vi "Save_Portfolio.vi"(7 "Config File path":path caption="Config File Path", 8 "error in (no error)":errorcluster caption="entrée d'erreur (pas d'erreur)", 10 "path":path, 11 "Portfolio in":refnum<class "Portfolio.lvclass">) -> (0 "error out":errorcluster caption="sortie d'erreur", 3 "Portfolio en sortie":refnum<class "Portfolio.lvclass"> caption="DNL_LabVIEW Object out")   [LabVIEW 2012, in "Portfolio.lvclass"]
uses:
  Portfolio.lvclass
  Stock/Stock Parameters.ctl
  controls/Currencies.ctl
  Portfolio.lvclass/Portfolio.ctl
  Stock/Stock.lvclass/Stock.ctl
  Operations/Operations.lvclass
  Exchanges/Exchanges.lvclass
  <vilib>/Utility/config.llb/NI_LVConfig.lvlib
  Stock/Stock.lvclass
panel:
  in  "Stocks":T1[](array[typedef])
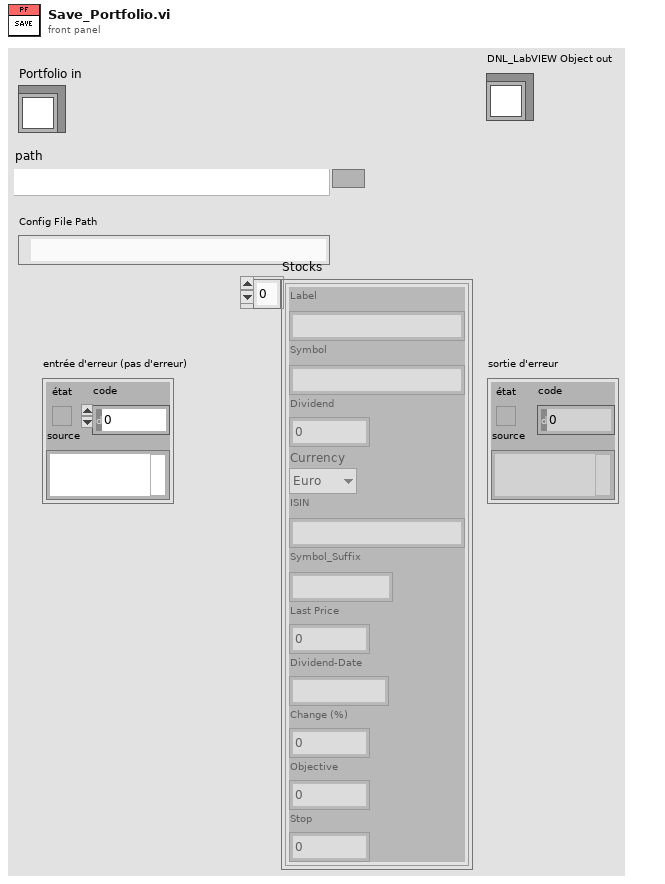
[diagram p1: front panel]
types:
  T1 = typedef "Stock.lvclass/Stock Parameters.ctl" = cluster{"Label":string, "Symbol":string, "Dividend":dbl, "Currency":T2, "ISIN":string, "Symbol_Suffix":string, "Last Price":dbl, "Dividend-Date":string, "Change (%)":dbl, "Objective":dbl, "Stop":dbl}
  T2 = typedef "Currencies.ctl" = enum16{"Euro", "Dollar", "Yen", "RIM", "CHF"}
  T3 = typedef "NI_LVConfig.lvlib/Config Data RefNum.ctl" = refnum<k1>
  T4 = typedef "Portfolio Parameters.ctl" = cluster{"Date":timestamp, "Name":string, "Cash":dbl, "Total":dbl, "Investissements":dbl, "Performance Totale (en %)":dbl, "Performance sur 1 an (en %)":dbl}
  T5 = typedef "Operation Parameters.ctl" = cluster{"Date":timestamp, "Operation Type":T6, "Amount":dbl, "Comment":string, "Currency":T2}
  T6 = typedef "Operation Type Enum.ctl" = enum16{"Coupons", "Dépot", "Retrait", "Intérêts", "Taxe"}
  T7 = typedef "Exchange Parameters.ctl" = cluster{"Date":timestamp, "Exchange Type":T8, "ISIN":string, "Label":string, "Price":dbl, "Qty":dbl, "Currency":T2, "Tax":dbl, "Comment":string, "PRU":dbl}
  T8 = typedef "Exchange.lvclass/Exchange Type Enum.ctl" = enum16{"ACHAT", "VENTE"}
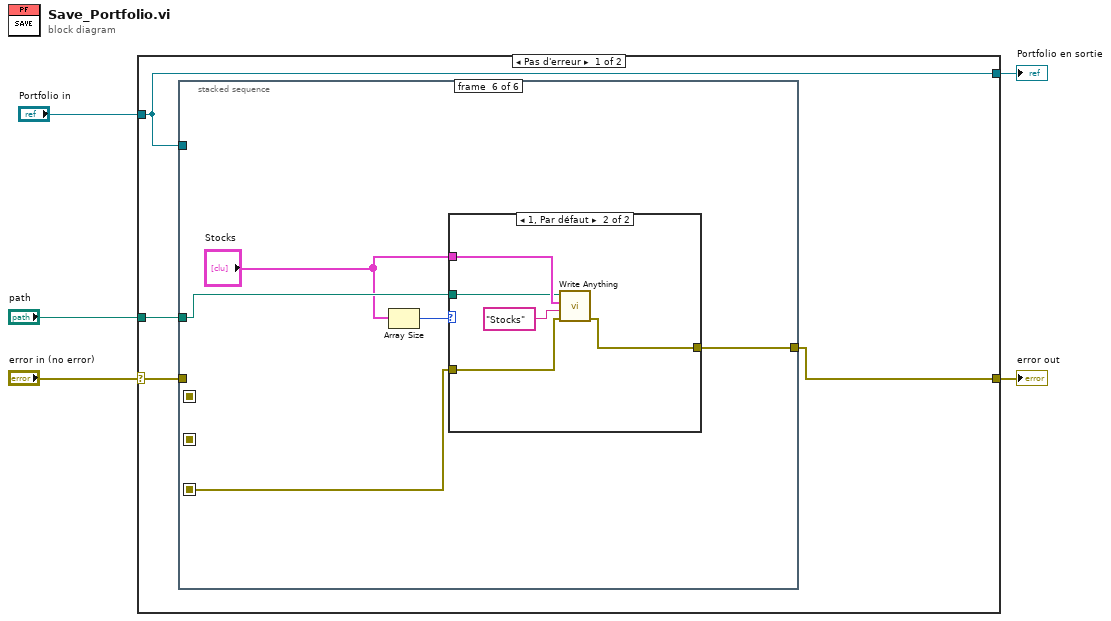
[diagram p0: block diagram]
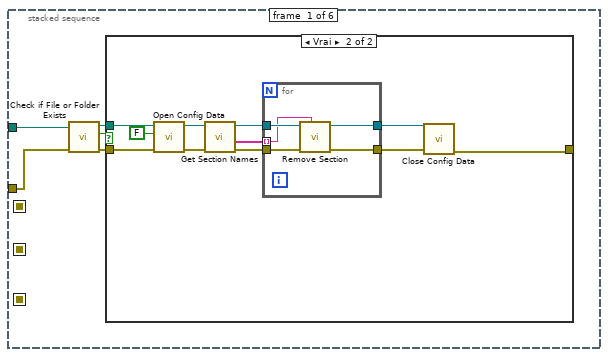
[diagram p2: hidden frame]
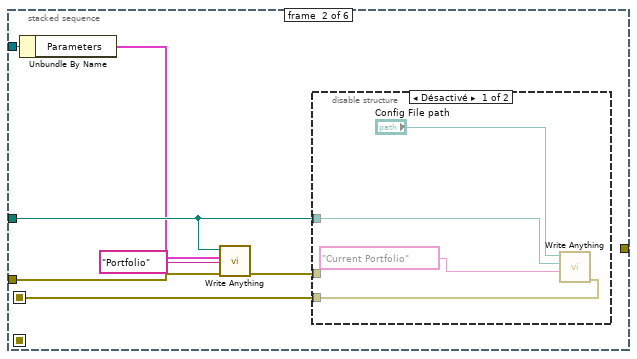
[diagram p4: hidden frame]
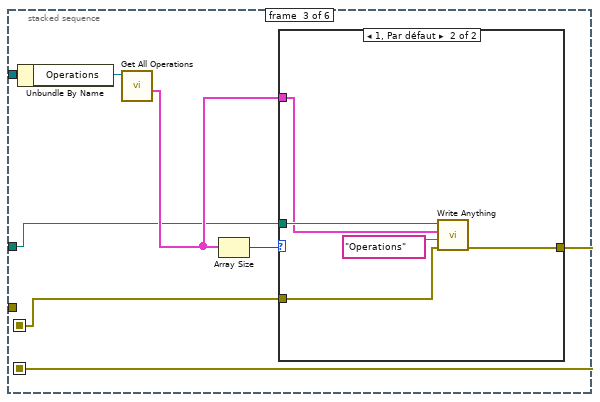
[diagram p6: hidden frame]
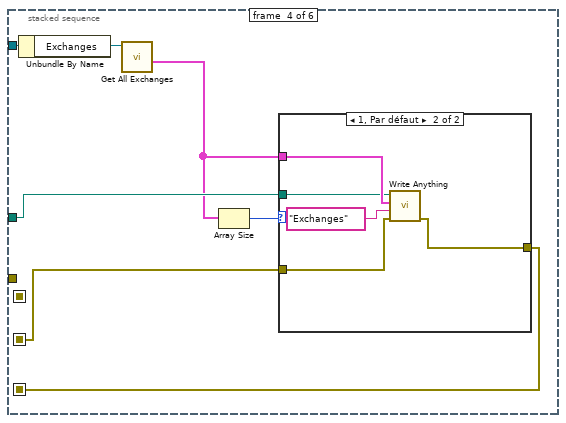
[diagram p8: hidden frame]
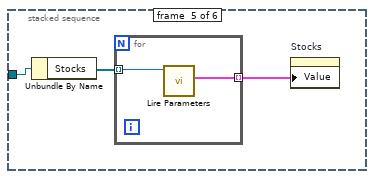
[diagram p10: hidden frame]
diagram:
  n1 = case shown="Pas d'erreur" "error in (no error)" {
    selector: "error in (no error)" -> [w9 w87]
    tunnel: [w7 w87] -> w4
    tunnel: [w6 w86] -> w2
    tunnel: "Portfolio in" -> [w6 w86]
    tunnel: "path" -> [w8 _]
    frame No Error {
      n2 = stacked-sequence {
        seq-local: [_ w37 _ _ _ _] -> [_ _ w45 _ _ _]
        seq-local: [_ _ w44 _ _ _] -> [_ _ _ w58 _ _]
        seq-local: [_ _ _ w57 _ _] -> [_ _ _ _ _ w77]
        tunnel: w6 -> [_ w38 w50 w63 w72 _]
        tunnel: w9 -> [w13 w34 _ _ _ _]
        tunnel: w8 -> [w14 w35 w46 w60 _ w78]
        tunnel: [_ _ _ _ _ w76] -> w7
        frame #0 {
          n3 = call <vilib>:"Check if File or Folder Exists.vi"("error in (no error)"=w13, "path"=w14) -> ("error out"=w12:errorcluster, "file or folder exists?"=w10:bool, "dup path"=w11:path)  [unwired: 7 in]
          n4 = case shown="Vrai" w10 {
            tunnel: w12 -> [w15 w26]
            tunnel: w11 -> [_ w25]
            tunnel: [w15 w16] -> _
            frame False {
            }
            frame True {
              n5 = call <vilib>:"Open Config Data.vi"("error in (no error)"=w26, "create file if necessary (T)"=FALSE, "configuration file path"=w25) -> ("error out"=w23:errorcluster, "refnum"=w22:T3)  [unwired: 6 in, 1 out]
              n6 = call <vilib>:"Get Section Names.vi"("error in (no error)"=w23, "refnum"=w22) -> ("error out"=w20:errorcluster, "section names"=w19:string[], "refnum out"=w21:T3)  [unwired: 7 in]
              n7 = for {
                tunnel: w21 -> [w31]
                tunnel: w20 -> [w30]
                tunnel: w19 -> [w29] mode=indexing
                tunnel: [w28] -> w17
                tunnel: [w27] -> w18
                n8 = call <vilib>:"Remove Section.vi"("section"=w29, "error in (no error)"=w30, "refnum"=w31) -> ("error out"=w28:errorcluster, "refnum out"=w27:T3)  [unwired: 6 in, 1 out]
              }
              n9 = call <vilib>:"Close Config Data.vi"("error in (no error)"=w17, "refnum"=w18) -> ("error out"=w16:errorcluster)  [unwired: 8 in, 1 out]
            }
          }
        }
        frame #1 {
          n10 = Unbundle By Name(w38) -> ("Parameters"=w32:T4)
          n11 = call "Write Anything.vi"("Error In"=w34, "Section Name (Name of \"Anything\")"="Portfolio" ("Instance Name"), "Anything"=w32, "Path (dialog)"=w35) -> ("Error Out"=w33:errorcluster)  [unwired: 7 in]
          n12 = disable-structure shown="Désactivé" {
            disable-tunnel: [w40 w43] -> w37
            disable-tunnel: w35 -> [w39 _]
            disable-tunnel: w33 -> [_ w43]
            frame Disabled {
              n13 = call "Write Anything.vi"("Section Name (Name of \"Anything\")"="Current Portfolio" ("button label"), "Anything"=w39, "Path (dialog)"="Config File path") -> ("Error Out"=w40:errorcluster)  [unwired: 8 in]
            }
            frame Enabled {
            }
          }
        }
        frame #2 {
          n14 = Unbundle By Name(w50) -> ("Operations"=w48:refnum<class "Operations.lvclass">)
          n15 = call "Get All Operations.vi"("Operations en entrée"=w48) -> ("Operations"=w47:T5[])  [unwired: 6 in, 4 out]
          n16 = Array Size(array=w47) -> (size(s)=w49:i32)
          n17 = case shown="1, Par défaut" w49 {
            tunnel: w47 -> [_ w52]
            tunnel: w46 -> [_ w56]
            tunnel: w45 -> [w51 w55]
            tunnel: [w51 w54] -> w44
            frame 0 {
            }
            frame 1, Default {
              n18 = call "Write Anything.vi"("Error In"=w55, "Section Name (Name of \"Anything\")"="Operations" ("Instance Name"), "Anything"=w52, "Path (dialog)"=w56) -> ("Error Out"=w54:errorcluster)  [unwired: 7 in]
            }
          }
        }
        frame #3 {
          n19 = Unbundle By Name(w63) -> ("Exchanges"=w61:refnum<class "Exchanges.lvclass">)
          n20 = call "Get All Exchanges.vi"("Exchanges en entrée"=w61) -> ("Exchanges"=w59:T7[])  [unwired: 6 in, 4 out]
          n21 = Array Size(array=w59) -> (size(s)=w62:i32)
          n22 = case shown="1, Par défaut" w62 {
            tunnel: w59 -> [_ w69]
            tunnel: w60 -> [_ w68]
            tunnel: w58 -> [w64 w67]
            tunnel: [w64 w66] -> w57
            frame 0 {
            }
            frame 1, Default {
              n23 = call "Write Anything.vi"("Error In"=w67, "Section Name (Name of \"Anything\")"="Exchanges" ("Instance Name"), "Anything"=w69, "Path (dialog)"=w68) -> ("Error Out"=w66:errorcluster)  [unwired: 7 in]
            }
          }
        }
        frame #4 {
          n24 = Unbundle By Name(w72) -> ("Stocks"=w71:refnum<class "Stock.lvclass">[])
          n25 = for {
            tunnel: w71 -> [w74] mode=indexing
            tunnel: [w73] -> w70 mode=indexing
            n26 = call "Lire Parameters.vi"("Stock en entrée"=w74) -> ("Parameters"=w73:T1)  [unwired: 9 in, 1 out]
          }
          n27 = property on="Stocks" class="Tabl (strict)"("Value"=w70) -> ()  [unwired: 2 in, 2 out]
        }
        frame #5 {
          n28 = Array Size(array="Stocks") -> (size(s)=w79:i32)
          n29 = case shown="1, Par défaut" w79 {
            tunnel: "Stocks" -> [_ w85]
            tunnel: w78 -> [_ w84]
            tunnel: w77 -> [w80 w83]
            tunnel: [w80 w82] -> w76
            frame 0 {
            }
            frame 1, Default {
              n30 = call "Write Anything.vi"("Error In"=w83, "Section Name (Name of \"Anything\")"="Stocks" ("Instance Name"), "Anything"=w85, "Path (dialog)"=w84) -> ("Error Out"=w82:errorcluster)  [unwired: 7 in]
            }
          }
        }
      }
    }
    frame Error {
    }
  }
  "error out" <- w4
  "Portfolio en sortie" <- w2
